vi "CycleGraphFitting.vi"(5 "samples":i32=3000, 7 "Grph_Dir":bool, 8 "L_Threshold":dbl, 9 "R_Threshold":dbl, 10 "width":i32=15, 11 "signal":waveform(dbl)) -> (2 "출력 웨이브폼 2":waveform(dbl)(graph) caption="Org", 3 "출력 웨이브폼":waveform(dbl)(graph) caption="Fitted")   [LabVIEW 2013]
uses:
  <vilib>/addons/Wavelet Analysis/application.llb/WA Multiscale Peak Detection (Waveform).vi
  <vilib>/Waveform/WDTOps.llb/WDT Waveform Duration DBL.vi
  <vilib>/Waveform/WDTOps.llb/WDT Get Waveform Subset DBL.vi
  <vilib>/addons/_Advanced Signal Processing/NI_AdvSigProcWA.lvlib
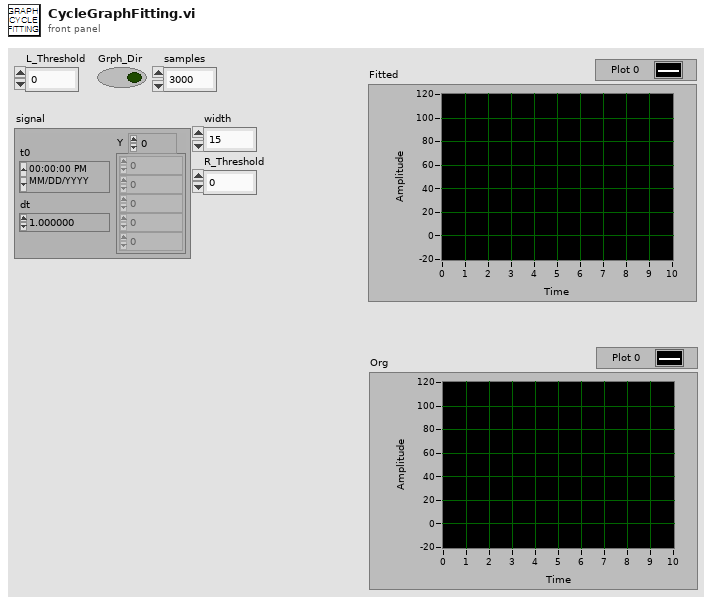
[diagram p1: front panel]
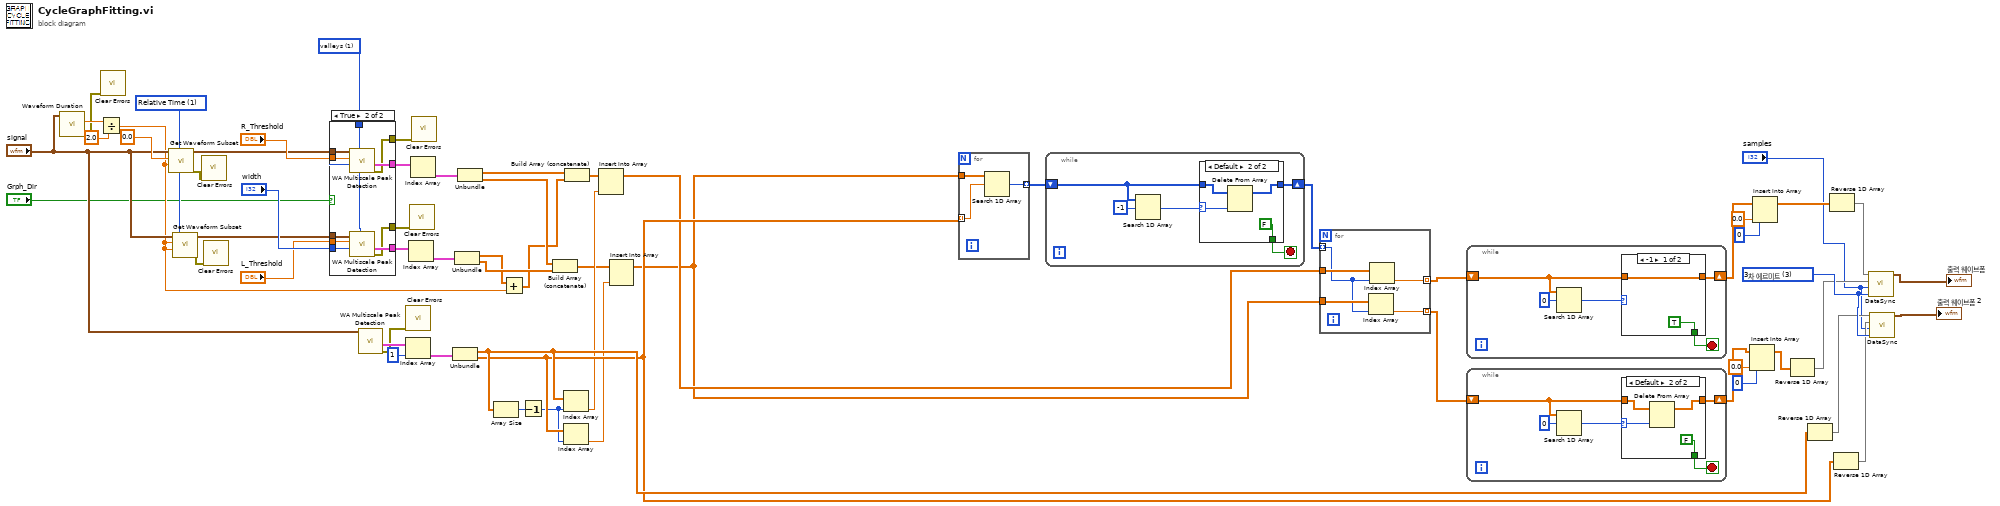
[diagram p0: block diagram]
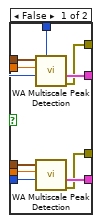
[diagram p2: hidden frame]
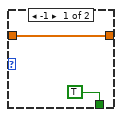
[diagram p3: hidden frame]
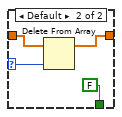
[diagram p4: hidden frame]
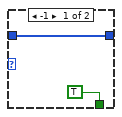
[diagram p5: hidden frame]
diagram:
  w29 = u16 1 items=["Samples", "Relative Time"] ("start/duration format")
  w52 = 3 items=["최근접", "선형", "스플라인", "3차 에르미트", "라그랑지"] ("method")
  w61 = u16 1 items=["peaks", "valleys"] ("peaks/valleys")
  n1 = call-poly <vilib>:"Waveform Duration.vi"("waveform in"="signal") -> ("error out"=w4:errorcluster, "duration"=w32:dbl)  [unwired: 8 in, 1 out]
  n2 = Divide(x=w32, y=2.0) -> (x/y=w22:dbl)
  n3 = call <vilib>:"Clear Errors.vi"("error in (no error)"=w4) -> ()  [unwired: 6 in, 1 out]
  n4 = call-poly <vilib>:"Get Waveform Subset.vi"("start/duration format"=w29, "duration"=w22, "start samples/time"=0.0, "waveform in"="signal") -> ("error out"=w6:errorcluster, "waveform out"=w28:waveform(dbl))  [unwired: 2 in, 2 out]
  n5 = call-poly <vilib>:"Get Waveform Subset.vi"("start/duration format"=w29, "duration"=w22, "start samples/time"=w22, "waveform in"="signal") -> ("error out"=w5:errorcluster, "waveform out"=w27:waveform(dbl))  [unwired: 2 in, 2 out]
  n6 = call <vilib>:"Clear Errors.vi"("error in (no error)"=w6) -> ()  [unwired: 6 in, 1 out]
  n7 = call <vilib>:"Clear Errors.vi"("error in (no error)"=w5) -> ()  [unwired: 6 in, 1 out]
  n8 = case shown="True" "Grph_Dir" {
    tunnel: w61 -> [w64 w81]
    tunnel: [w71 w80] -> w60
    tunnel: [w70 w79] -> w53
    tunnel: "width" -> [w69 w78]
    tunnel: "R_Threshold" -> [w68 w77]
    tunnel: "L_Threshold" -> [w67 w76]
    tunnel: w28 -> [w66 w75]
    tunnel: w27 -> [w65 w74]
    tunnel: [w63 w73] -> w3
    tunnel: [w62 w72] -> w2
    frame False {
      n9 = call-poly <vilib>:"WA Multiscale Peak Detection.vi"("peaks/valleys"=w64, "width"=w69, "threshold"=w68, "signal"=w66) -> ("error out"=w63:errorcluster, "peak plot"=w70:cluster{"Ramp Pattern":dbl[], "X":dbl[]}[])  [unwired: 3 in, 3 out]
      n10 = call-poly <vilib>:"WA Multiscale Peak Detection.vi"("width"=w69, "threshold"=w67, "signal"=w65) -> ("error out"=w62:errorcluster, "peak plot"=w71:cluster{"Ramp Pattern":dbl[], "X":dbl[]}[])  [unwired: 4 in, 3 out]
    }
    frame True {
      n11 = call-poly <vilib>:"WA Multiscale Peak Detection.vi"("width"=w78, "threshold"=w77, "signal"=w75) -> ("error out"=w73:errorcluster, "peak plot"=w79:cluster{"Ramp Pattern":dbl[], "X":dbl[]}[])  [unwired: 4 in, 3 out]
      n12 = call-poly <vilib>:"WA Multiscale Peak Detection.vi"("peaks/valleys"=w81, "width"=w78, "threshold"=w76, "signal"=w74) -> ("error out"=w72:errorcluster, "peak plot"=w80:cluster{"Ramp Pattern":dbl[], "X":dbl[]}[])  [unwired: 3 in, 3 out]
    }
  }
  n13 = call-poly <vilib>:"WA Multiscale Peak Detection.vi"("signal"="signal") -> ("error out"=w1:errorcluster, "peak plot"=w25:cluster{"Ramp Pattern":dbl[], "X":dbl[]}[])  [unwired: 6 in, 3 out]
  n14 = call <vilib>:"Clear Errors.vi"("error in (no error)"=w1) -> ()  [unwired: 6 in, 1 out]
  n15 = Index Array(array=w25, index=1) -> (element=w23:cluster{"Ramp Pattern":dbl[], "X":dbl[]})
  n16 = Index Array(array=w60) -> (element=w54:cluster{"Ramp Pattern":dbl[], "X":dbl[]})  [unwired: 1 in]
  n17 = call <vilib>:"Clear Errors.vi"("error in (no error)"=w2) -> ()  [unwired: 6 in, 1 out]
  n18 = Index Array(array=w53) -> (element=w59:cluster{"Ramp Pattern":dbl[], "X":dbl[]})  [unwired: 1 in]
  n19 = call <vilib>:"Clear Errors.vi"("error in (no error)"=w3) -> ()  [unwired: 6 in, 1 out]
  n20 = Unbundle(w23) -> ("Ramp Pattern"=w17:dbl[], "X"=w16:dbl[])
  n21 = Unbundle(w54) -> ("Ramp Pattern"=w20:dbl[], "X"=w21:dbl[])
  n22 = Unbundle(w59) -> ("Ramp Pattern"=w34:dbl[], "X"=w35:dbl[])
  n23 = Array Size(array=w17) -> (size(s)=w18:i32)
  n24 = Add(x=w20, y=w22) -> (x+y=w19:dbl[])
  n25 = Decrement(x=w18) -> (x-1=w15:i32)
  n26 = Build Array (concatenate)(w35, w21) -> (w11:dbl[])
  n27 = Index Array(array=w17, index=w15) -> (element=w13:dbl)
  n28 = Index Array(array=w16, index=w15) -> (element=w10:dbl)
  n29 = Build Array (concatenate)(w34, w19) -> (w14:dbl[])
  n30 = Insert Into Array(array=w14, new element=w13) -> (w12:dbl[])  [unwired: 1 in]
  n31 = Insert Into Array(array=w11, new element=w10) -> (w9:dbl[])  [unwired: 1 in]
  n32 = for {
    tunnel: w16 -> [w83] mode=indexing
    tunnel: w9 -> [w84]
    tunnel: [w82] -> w58 mode=indexing
    n33 = Search 1D Array(1D array=w84, element=w83) -> (index of element=w82:i32)  [unwired: 1 in]
  }
  n34 = while {
    shift-right: [w89] -> w57
    shift-left: w58 -> [w88]
    stop <- w86 stop-if-true
    n35 = Search 1D Array(1D array=w88, element=-1) -> (index of element=w87:i32)  [unwired: 1 in]
    n36 = case shown="Default" w87 {
      selector: w87 -> [_ w93]
      tunnel: w88 -> [w91 w95]
      tunnel: [w91 w94] -> w89
      tunnel: [TRUE FALSE] -> w86
      frame -1 {
      }
      frame Default {
        n37 = Delete From Array(array=w95, index=w93) -> (array with subset deleted=w94:i32[])  [unwired: 1 in, 1 out]
      }
    }
  }
  n38 = for {
    tunnel: w57 -> [w98] mode=indexing
    tunnel: w12 -> [w100]
    tunnel: w9 -> [w99]
    tunnel: [w97] -> w56 mode=indexing
    tunnel: [w96] -> w55 mode=indexing
    n39 = Index Array(array=w99, index=w98) -> (element=w96:dbl)
    n40 = Index Array(array=w100, index=w98) -> (element=w97:dbl)
  }
  n41 = while {
    shift-right: [w105] -> w50
    shift-left: w56 -> [w104]
    stop <- w102 stop-if-true
    n42 = Search 1D Array(1D array=w104, element=0) -> (index of element=w103:i32)  [unwired: 1 in]
    n43 = case shown="-1" w103 {
      selector: w103 -> [_ w109]
      tunnel: w104 -> [w107 w111]
      tunnel: [w107 w110] -> w105
      tunnel: [TRUE FALSE] -> w102
      frame -1 {
      }
      frame Default {
        n44 = Delete From Array(array=w111, index=w109) -> (array with subset deleted=w110:dbl[])  [unwired: 1 in, 1 out]
      }
    }
  }
  n45 = while {
    shift-right: [w116] -> w48
    shift-left: w55 -> [w115]
    stop <- w113 stop-if-true
    n46 = Search 1D Array(1D array=w115, element=0) -> (index of element=w114:i32)  [unwired: 1 in]
    n47 = case shown="Default" w114 {
      selector: w114 -> [_ w120]
      tunnel: w115 -> [w118 w122]
      tunnel: [w118 w121] -> w116
      tunnel: [TRUE FALSE] -> w113
      frame -1 {
      }
      frame Default {
        n48 = Delete From Array(array=w122, index=w120) -> (array with subset deleted=w121:dbl[])  [unwired: 1 in, 1 out]
      }
    }
  }
  n49 = Insert Into Array(array=w48, index=0, new element=0.0 ("new element/subarray")) -> (w42:dbl[])
  n50 = Insert Into Array(array=w50, index=0, new element=0.0 ("new element/subarray")) -> (w44:dbl[])
  n51 = Reverse 1D Array(array=w42) -> (reversed array=w41:dbl[])
  n52 = Reverse 1D Array(array=w17) -> (reversed array=w40:dbl[])
  n53 = Reverse 1D Array(array=w44) -> (reversed array=w43:dbl[])
  n54 = Reverse 1D Array(array=w16) -> (reversed array=w39:dbl[])
  n55 = call "DataSync.vi"("method"=w52, "samples"="samples", "Y"=w41, "X"=w43) -> ("출력 웨이브폼"=→"출력 웨이브폼":waveform(dbl))  [unwired: 5 in, 2 out]
  n56 = call "DataSync.vi"("method"=w52, "samples"="samples", "Y"=w39, "X"=w40) -> ("출력 웨이브폼"=→"출력 웨이브폼 2":waveform(dbl))  [unwired: 5 in, 2 out]
